vi "Check_FGV.vi"(8 "Error In":errorcluster, 11 "Action":T1) -> (0 "Error Out":errorcluster, 1 "Dot String":string, 2 "+- Out":string, 3 "Number ?":bool, 5 "Shift ?":bool)   [LabVIEW 2021, in "Signal.lvlib"]
doc: "This FGV is used to check if \" . \" or \" +/-\" is clicked. If the the controls are clicked odd number of times the output will be decimal and \" - \" respectively and vice versa ."
uses:
  Signal.lvlib
  Tipski Definicii/check.ctl
panel:
  # "Output"
  # "Input"
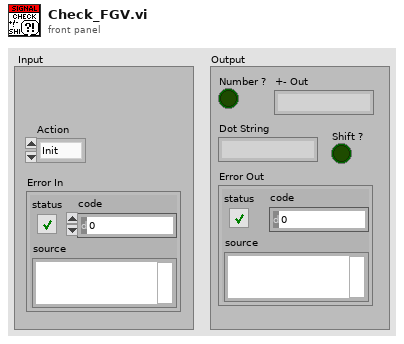
[diagram p1: front panel]
types:
  T1 = typedef "check.ctl" = enum16{"Init", "Add dot", "Add +", "Add Shift", "Check", "Reset", "Reset Shift"}
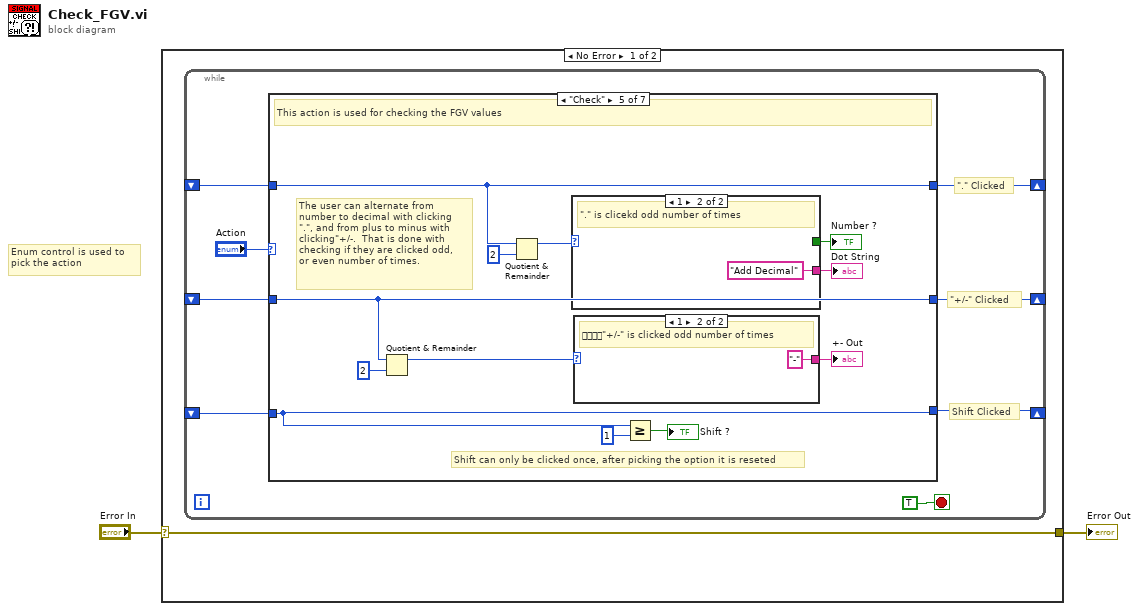
[diagram p0: block diagram]
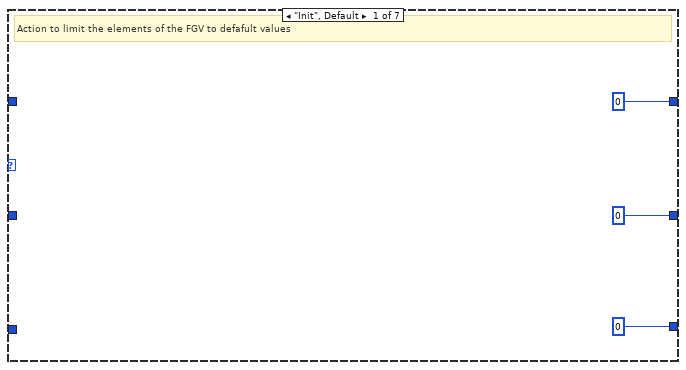
[diagram p2: hidden frame]
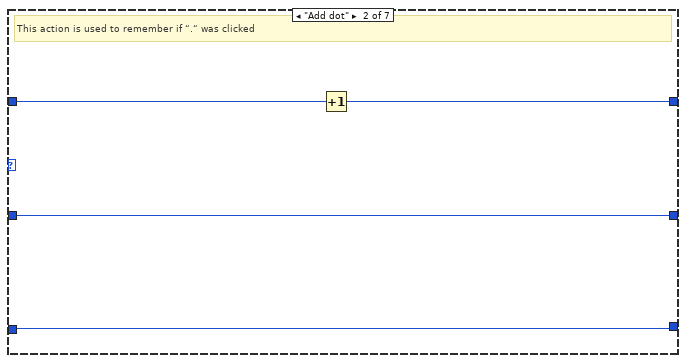
[diagram p3: hidden frame]
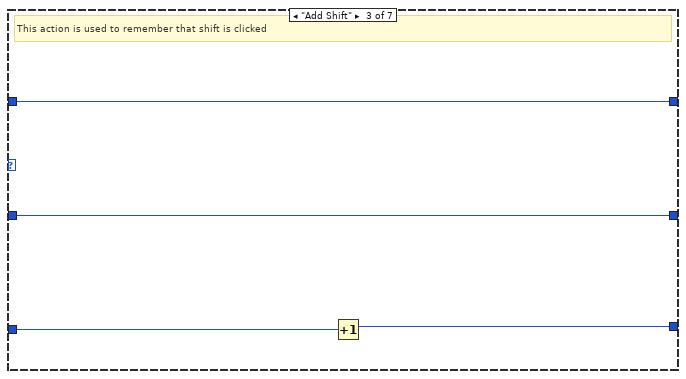
[diagram p4: hidden frame]
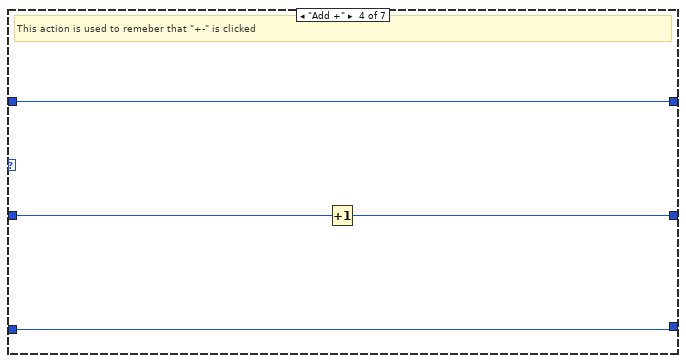
[diagram p5: hidden frame]
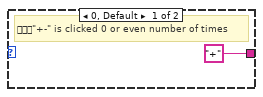
[diagram p6: hidden frame]
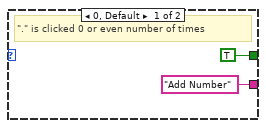
[diagram p7: hidden frame]
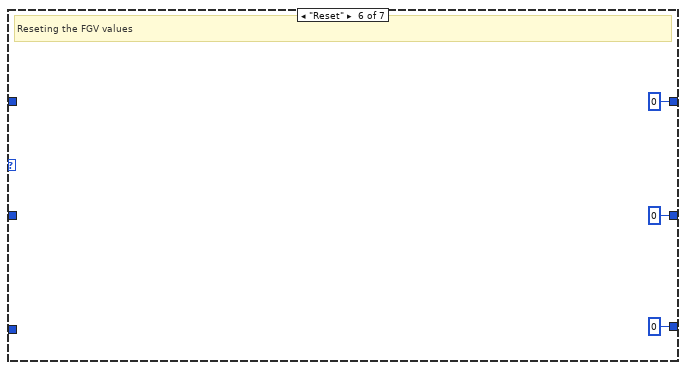
[diagram p8: hidden frame]
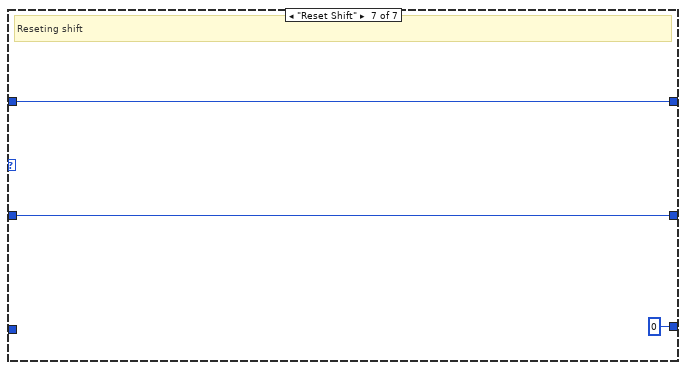
[diagram p9: hidden frame]
diagram:
  # "Enum control is used to \npick the action"
  n1 = case shown="No Error" "Error In" {
    selector: "Error In" -> [w3 w50]
    tunnel: [w3 w50] -> w1
    frame No Error {
      n2 = while {
        shift-right: [w9] -> _
        shift-left: _ -> [w8]
        shift-right: [w7] -> _
        shift-left: _ -> [w6]
        shift-right: [w5] -> _
        shift-left: _ -> [w4]
        stop <- TRUE stop-if-true
        # "Shift Clicked"
        # "\"+/-\" Clicked"
        # "\".\" Clicked"
        n3 = case shown="\"Check\"" "Action" {
          tunnel: [0 w17 w22 w26 w38 0 w49] -> w9
          tunnel: w8 -> [_ w18 w22 w26 w38 _ w49]
          tunnel: [0 w16 w21 w24 w33 0 w48] -> w7
          tunnel: w6 -> [_ w16 w21 w25 w33 _ w48]
          tunnel: [0 w15 w19 w23 w28 0 0] -> w5
          tunnel: w4 -> [_ w15 w20 w23 w28 _ _]
          frame "Init", Default {
            # "Action to limit the elements of the FGV to defafult values"
          }
          frame "Add dot" {
            # "This action is used to remember if “.“ was clicked"
            n4 = Increment(x=w18) -> (x+1=w17:i32)
          }
          frame "Add Shift" {
            # "This action is used to remember that shift is clicked"
            n5 = Increment(x=w20) -> (x+1=w19:i32)
          }
          frame "Add +" {
            # "This action is used to remeber that \"+-\" is clicked"
            n6 = Increment(x=w25) -> (x+1=w24:i32)
          }
          frame "Check" {
            # "Shift can only be clicked once, after picking the option it is reseted"
            # "The user can alternate from \nnumber to decimal with clicking\n\".\", and from plus to minus with \nclicking\"+/-.  That is done with\nchecking if they are clicked odd,\nor even number of times."
            # "This action is used for checking the FGV values"
            n7 = Quotient & Remainder(x=w33, y=2) -> (x-y*floor(x/y)=w32:i32)  [unwired: 1 out]
            n8 = Quotient & Remainder(x=w38, y=2) -> (x-y*floor(x/y)=w36:i32)  [unwired: 1 out]
            n9 = case shown="1" w36 {
              tunnel: [TRUE _] -> w35
              tunnel: ["Add Number" "Add Decimal"] -> w30
              frame 0, Default {
                # "\".\" is clicked 0 or even number of times"
              }
              frame 1 {
                # "\".\" is clicekd odd number of times"
              }
            }
            "Number ?" <- w35
            "Dot String" <- w30
            n10 = case shown="1" w32 {
              tunnel: ["+" "-"] -> w31
              frame 0, Default {
                # "\"+-\" is clicked 0 or even number of times"
              }
              frame 1 {
                # "\"+/-\" is clicked odd number of times"
              }
            }
            "+- Out" <- w31
            n11 = Greater Or Equal?(x=w28, y=1) -> (x >= y?=→"Shift ?":bool)
          }
          frame "Reset" {
            # "Reseting the FGV values"
          }
          frame "Reset Shift" {
            # "Reseting shift"
          }
        }
      }
    }
    frame Error {
    }
  }
  "Error Out" <- w1
